vi "Get Task.vi"(8 "error in (no error)":errorcluster, 11 "DAQmx Base CFG in":refnum<class "DAQmx Base CFG.lvclass">) -> (0 "error out":errorcluster, 2 "Task":refnum<k21>, 3 "DAQmx Base CFG out":refnum<class "DAQmx Base CFG.lvclass">)   [LabVIEW 2023, in "DAQmx Base CFG.lvclass"]
uses:
  DAQmx Base CFG.lvclass
  DAQmx Base CFG.lvclass/DAQmx Base CFG.ctl
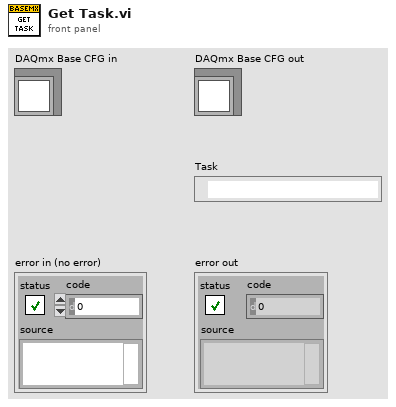
[diagram p1: front panel]
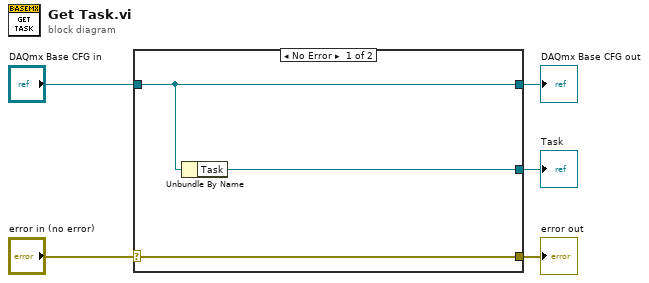
[diagram p0: block diagram]
diagram:
  n1 = case shown="No Error" "error in (no error)" {
    selector: "error in (no error)" -> [w8 w9]
    tunnel: [w8 w9] -> w4
    tunnel: [w7 w10] -> w2
    tunnel: "DAQmx Base CFG in" -> [w7 w10]
    tunnel: [w6 _] -> w1
    frame No Error {
      n2 = Unbundle By Name(w7) -> ("Task"=w6:refnum<k21>)
    }
    frame Error {
    }
  }
  "error out" <- w4
  "DAQmx Base CFG out" <- w2
  "Task" <- w1
